vi "start control.vi"() -> (1 "error out":errorcluster, 2 "reference out":refnum<k7>)   [LabVIEW 2011]
panel:
  in  "error in (no error)":errorcluster
  in  "MG17Motor":refnum<k7>(container)
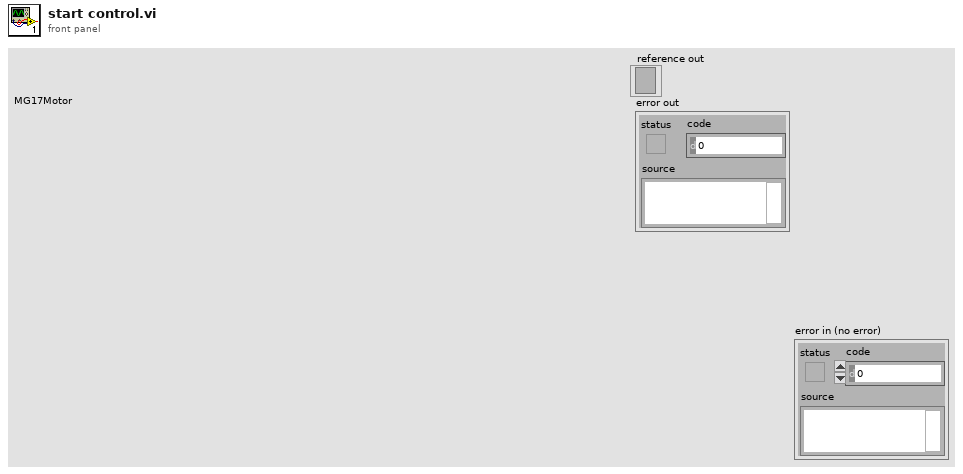
[diagram p1: front panel]
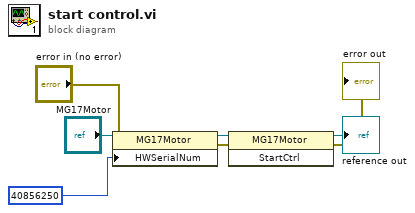
[diagram p0: block diagram]
diagram:
  n1 = property class="MG17Motor"(reference="MG17Motor", error in="error in (no error)", "HWSerialNum"=40856250) -> (reference out=w5:refnum<k7>, error out=w3:errorcluster)
  n2 = invoke class="MG17Motor" method="StartCtrl"(reference=w5, error in=w3) -> (reference out=→"reference out":refnum<k7>, error out=→"error out":errorcluster)  [unwired: 1 in, 1 out]
